vi "FlagIsOn.vi"(8 "error in (no error)":errorcluster, 10 "Flag to Check":T1, 11 "Room in":refnum<class "Room.lvclass">) -> (0 "error out":errorcluster, 2 "Flag Is On":bool)   [LabVIEW 2015, in "DatabaseApi.lvlib"]
uses:
  DatabaseApi.lvlib
  LVClasses/Room/Room.lvclass
  LVClasses/Flags/ColorEnum.ctl
  LVClasses/Room/Room.lvclass/Room.ctl
  LVClasses/Flags/Flags.lvclass/Flags.ctl
  LVClasses/Flags/Flags.lvclass
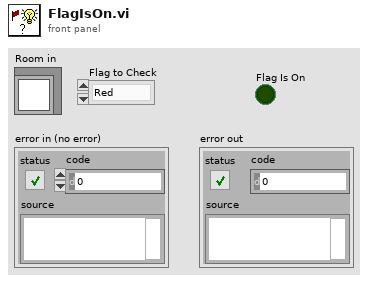
[diagram p1: front panel]
types:
  T1 = typedef "Flags.lvclass/ColorEnum.ctl" = enum8{"Red", "Blue", "Green", "Yellow"}
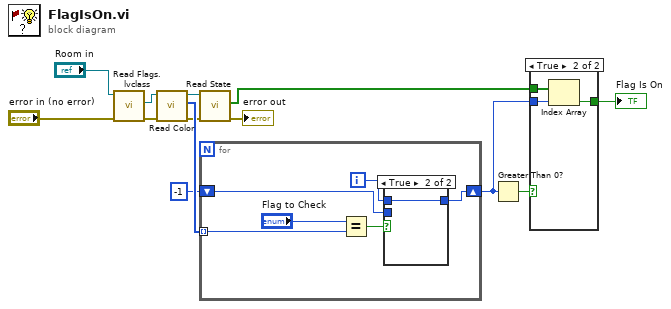
[diagram p0: block diagram]
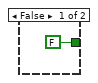
[diagram p2: hidden frame]
diagram:
  n1 = call "Read Flags.lvclass.vi"("error in (no error)"="error in (no error)", "Room in"="Room in") -> ("error out"=w12:errorcluster, "Flags.lvclass"=w11:refnum<class "Flags.lvclass">)  [unwired: 7 in, 1 out]
  n2 = call "Read Color.vi"("error in (no error)"=w12, "Flags in"=w11) -> ("error out"=w10:errorcluster, "Color"=w13:T1[], "Flags out"=w5:refnum<class "Flags.lvclass">)  [unwired: 7 in]
  n3 = call "Read State.vi"("error in (no error)"=w10, "Flags in"=w5) -> ("error out"=→"error out":errorcluster, "State"=w3:bool[])  [unwired: 7 in, 1 out]
  n4 = for {
    tunnel: w13 -> [w19] mode=indexing
    shift-right: [w15] -> w2
    shift-left: -1 -> [w14]
    i -> [w16]
    n5 = Equal?(x="Flag to Check", y=w19) -> (x = y?=w17:bool)
    n6 = case shown="True" w17 {
      tunnel: [w20 w21] -> w15
      tunnel: w16 -> [_ w21]
      tunnel: w14 -> [w20 _]
      frame False {
      }
      frame True {
      }
    }
  }
  n7 = Greater Than 0?(x=w2) -> (x > 0?=w4:bool)
  n8 = case shown="True" w4 {
    tunnel: w3 -> [_ w25]
    tunnel: w2 -> [_ w24]
    tunnel: [FALSE ("Boolean") w23] -> w1
    frame False {
    }
    frame True {
      n9 = Index Array(array=w25, index=w24) -> (element=w23:bool)
    }
  }
  "Flag Is On" <- w1
